vi "Sequence of Chebyshev Approximations.vi"() -> ()   [LabVIEW 2023]
doc: "Evaluates and graphs a one-variable equation. This example also calculates and graphs the Chebyshev approximation of the equation."
uses:
  <vilib>/gmath/NI_Gmath.lvlib
panel:
  in  "Error Message":string="Invalid 'function' input."
  in  "Stop":bool
  in  "Tab Control":enum32{"Example", "Theory"}(tab)
  out "error text":string
  in  "function":string="sin(x)-cos(sinc(x*x))"
  in  "start":dbl format="%#.6g"
  in  "end":dbl=7.0 format="%#.6g"
  in  "# of points":u32=56
  in  "order":u32=14
  out "XY Graph":cluster{"X":dbl[], "Y":dbl[]}[](graph)
  # "Overview: Demonstrates the use of the Chebyshev Approximation VI to approximate 1D functions by Chebyshev polynomials.\nRequirements: LabVIEW Full Development System\nInstructions:\n1. Run the VI.\n2. Change the value of order.\n3. View the result of Chebyshev Approximation in the graph.\n4. Click Stop to stop the VI."
  # "Sequence of Chebyshev Polynomials"
  # "The approximation of given functions by special sets of well-defined functions is a standard problem. In some sense the approximation of given functions by Chebyshev polynomials is the most efficient. If the interval of interest is [-1,1] the Chebyshev polynomials are defined by:\n\nTn(x) = cos (n arccos x)\n\nA given function f(x) can be approximated by:"
  # ", where"
  # "with"
  # "The VI demonstrates the accuracy of Chebyshev approximations for general intervals [a,b] and for symbolically given functions."
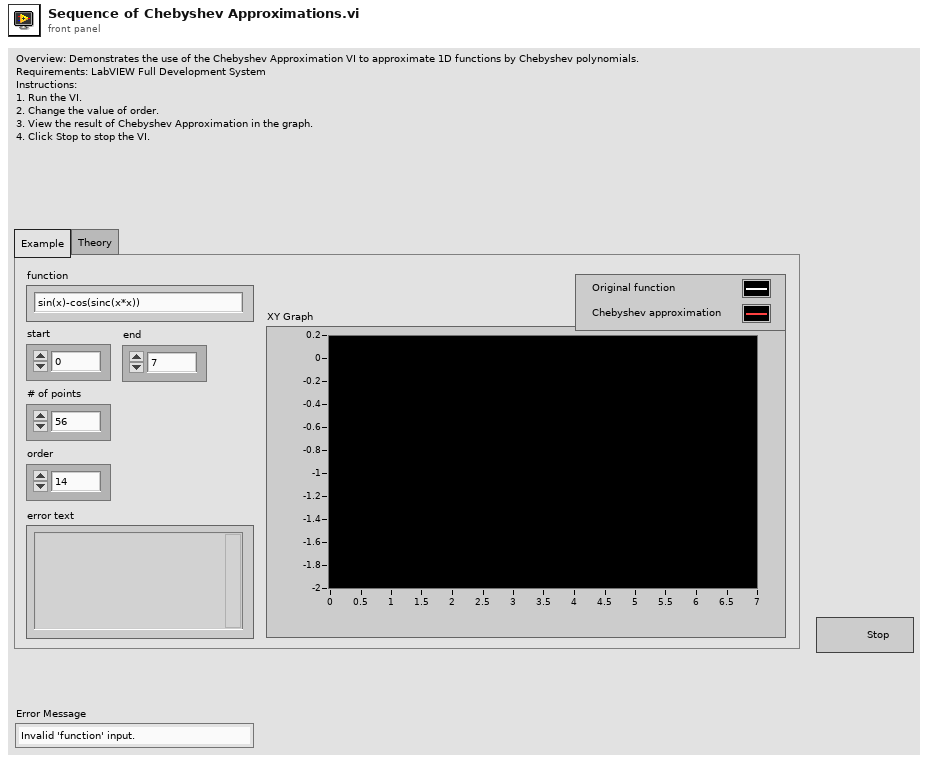
[diagram p1: front panel]
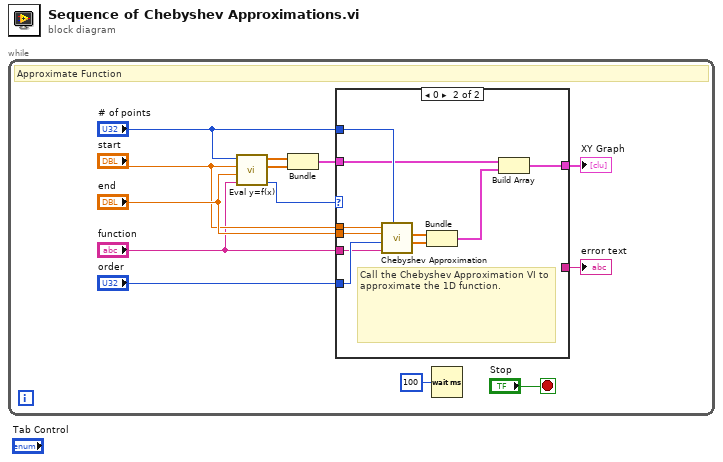
[diagram p0: block diagram]
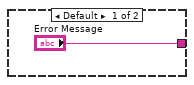
[diagram p2: hidden frame]
diagram:
  n1 = while {
    stop <- "Stop" stop-if-true
    # "Approximate Function"
    n2 = call <vilib>:"Eval y=f(x).vi"("formula"="function", "end"="end", "start"="start", "number of points"="# of points") -> ("error"=w1:i32, "Y Values"=w10:dbl[], "X Values"=w9:dbl[])  [unwired: 1 out]
    n3 = Bundle("X Values"=w9, "Y Values"=w10) -> (w11:cluster{"X Values":dbl[], "Y Values":dbl[]})  [unwired: 1 in]
    n4 = case shown="0" w1 {
      tunnel: "# of points" -> [_ w24]
      tunnel: "start" -> [_ w23]
      tunnel: "end" -> [_ w22]
      tunnel: "order" -> [_ w21]
      tunnel: "function" -> [_ w20]
      tunnel: w11 -> [_ w17]
      tunnel: [_ w15] -> w4
      tunnel: ["Error Message" _] -> w2
      frame Default {
      }
      frame 0 {
        # "Call the Chebyshev Approximation VI to approximate the 1D function."
        n5 = call <vilib>:"Chebyshev Approximation.vi"("number of points"=w24, "formula"=w20, "order"=w21, "end"=w22, "start"=w23) -> ("Y"=w18:dbl[], "X"=w19:dbl[])  [unwired: 2 out]
        n6 = Bundle("X"=w19, "Y"=w18) -> (w16:cluster{"X":dbl[], "Y":dbl[]})  [unwired: 1 in]
        n7 = Build Array(w17, w16) -> (w15:cluster{"X":dbl[], "Y":dbl[]}[])
      }
    }
    "error text" <- w2
    "XY Graph" <- w4
    n8 = Wait (ms)(milliseconds to wait=u32 100) -> ()  [unwired: 1 out]
  }
